vi "save_data.vi"(0 "Experiment Indicator":string, 2 "Date array":string[](array[string]), 3 "Scan direction":i32, 4 "Data Array":dbl[][](array[numeric]), 6 "Username":string, 7 "Stabilisation time (ms)":dbl, 8 "Cell details cluster":T1={"Cell Position"=16, "Cell Label"="", "Pixel to measure"=0, "Area (cm^2)"=0.126, "Variable"="", "Variable value"="", "Scan settings in queue"=0, "Light or dark"="", "Measurement type"=""} {"Pixel to measure" items=["All", "1", "2", "3", "4", "5", "6", "7", "8"]}, 10 "Measurement Delay (ms)":dbl=1.0, 11 "Stabilisation level \n(A or V depending on mode)":dbl=-1.4, 13 "Stabilisation Data":dbl[][](array[numeric])) -> (14 "Master Log":string[][](table), 15 "File path for master log":path, 17 "File path for JV data":path, 18 "File path for JV image":path)   [LabVIEW 2016]
uses:
  <vilib>/Utility/file.llb/Write Delimited Spreadsheet (string).vi
  <vilib>/Utility/file.llb/Read Delimited Spreadsheet (string).vi
  <vilib>/Analysis/NI_AALPro.lvlib
panel:
  out "Vmp":dbl
  out "PCE":dbl
  out "FF":dbl
  out "Voc":dbl
  out "Jsc":dbl
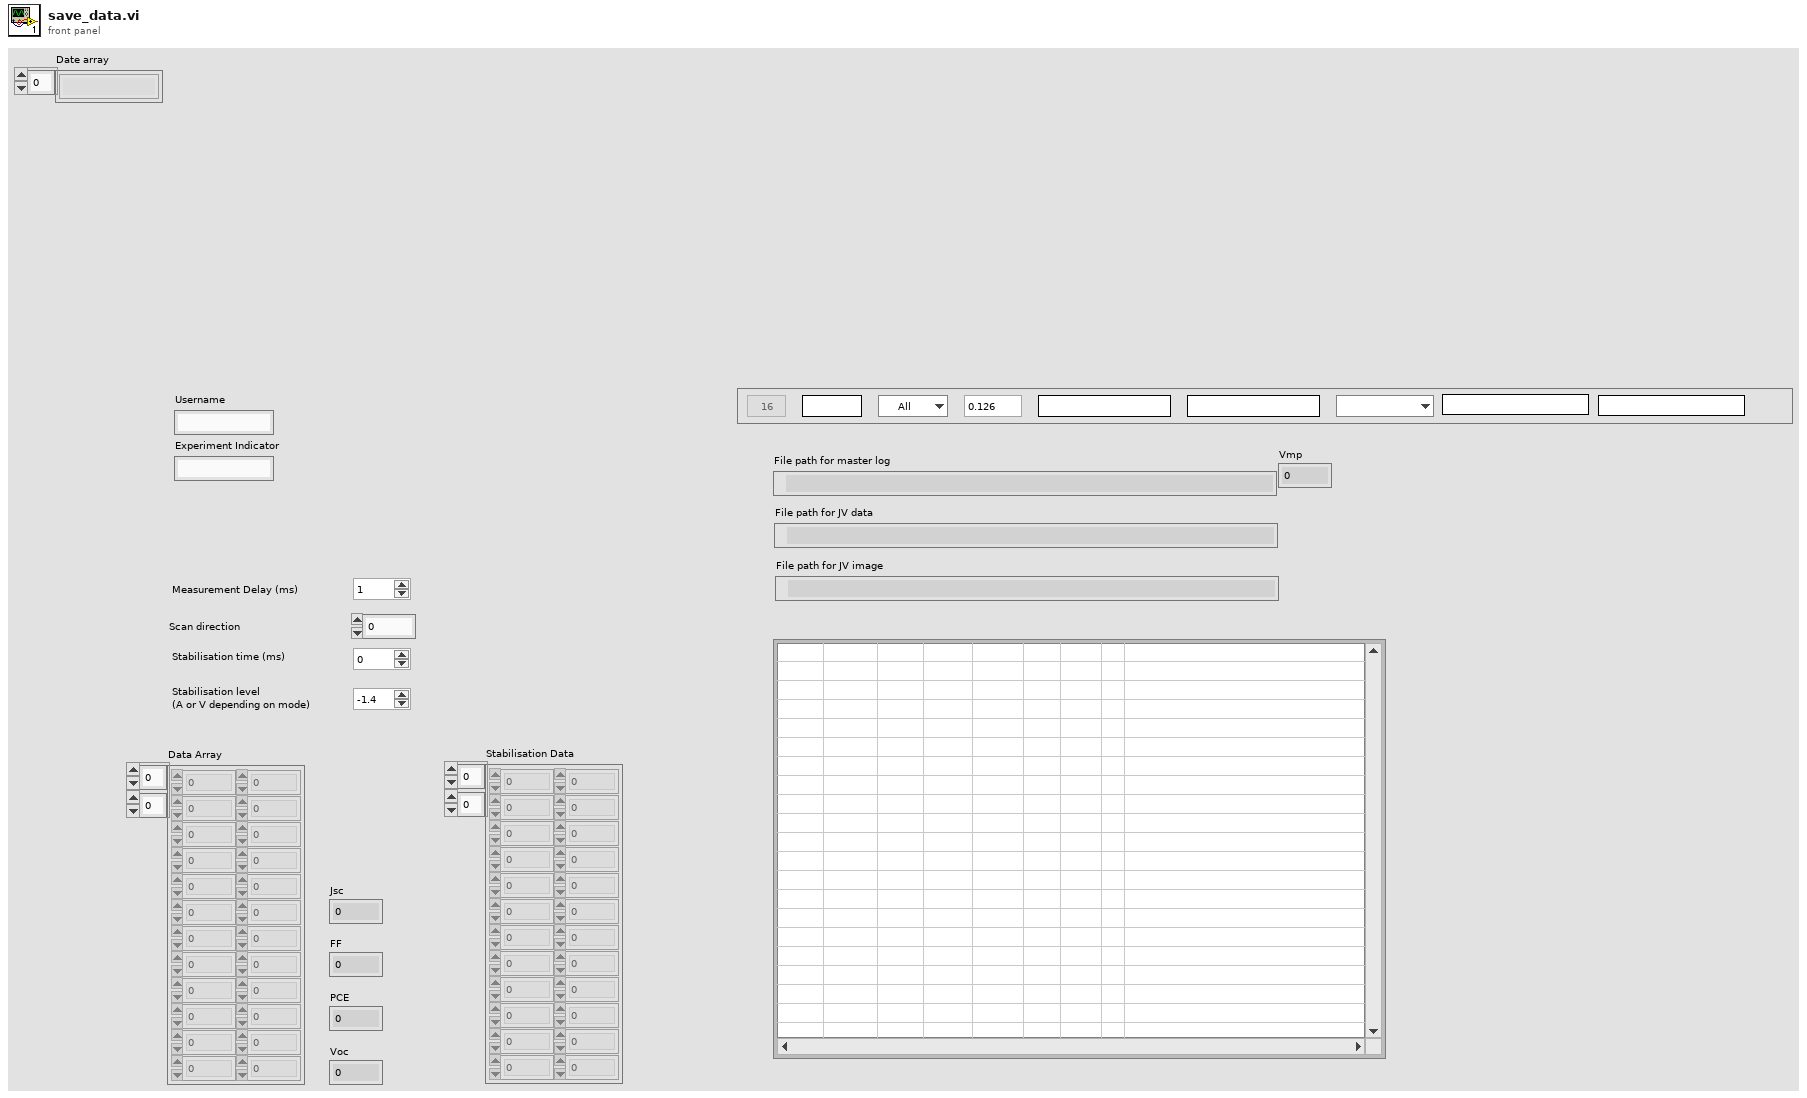
[diagram p1: front panel]
types:
  T1 = cluster{"Cell Position":i32, "Cell Label":string, "Pixel to measure":u16, "Area (cm^2)":dbl, "Variable":string, "Variable value":string, "Scan settings in queue":u16, "Light or dark":string, "Measurement type":string}
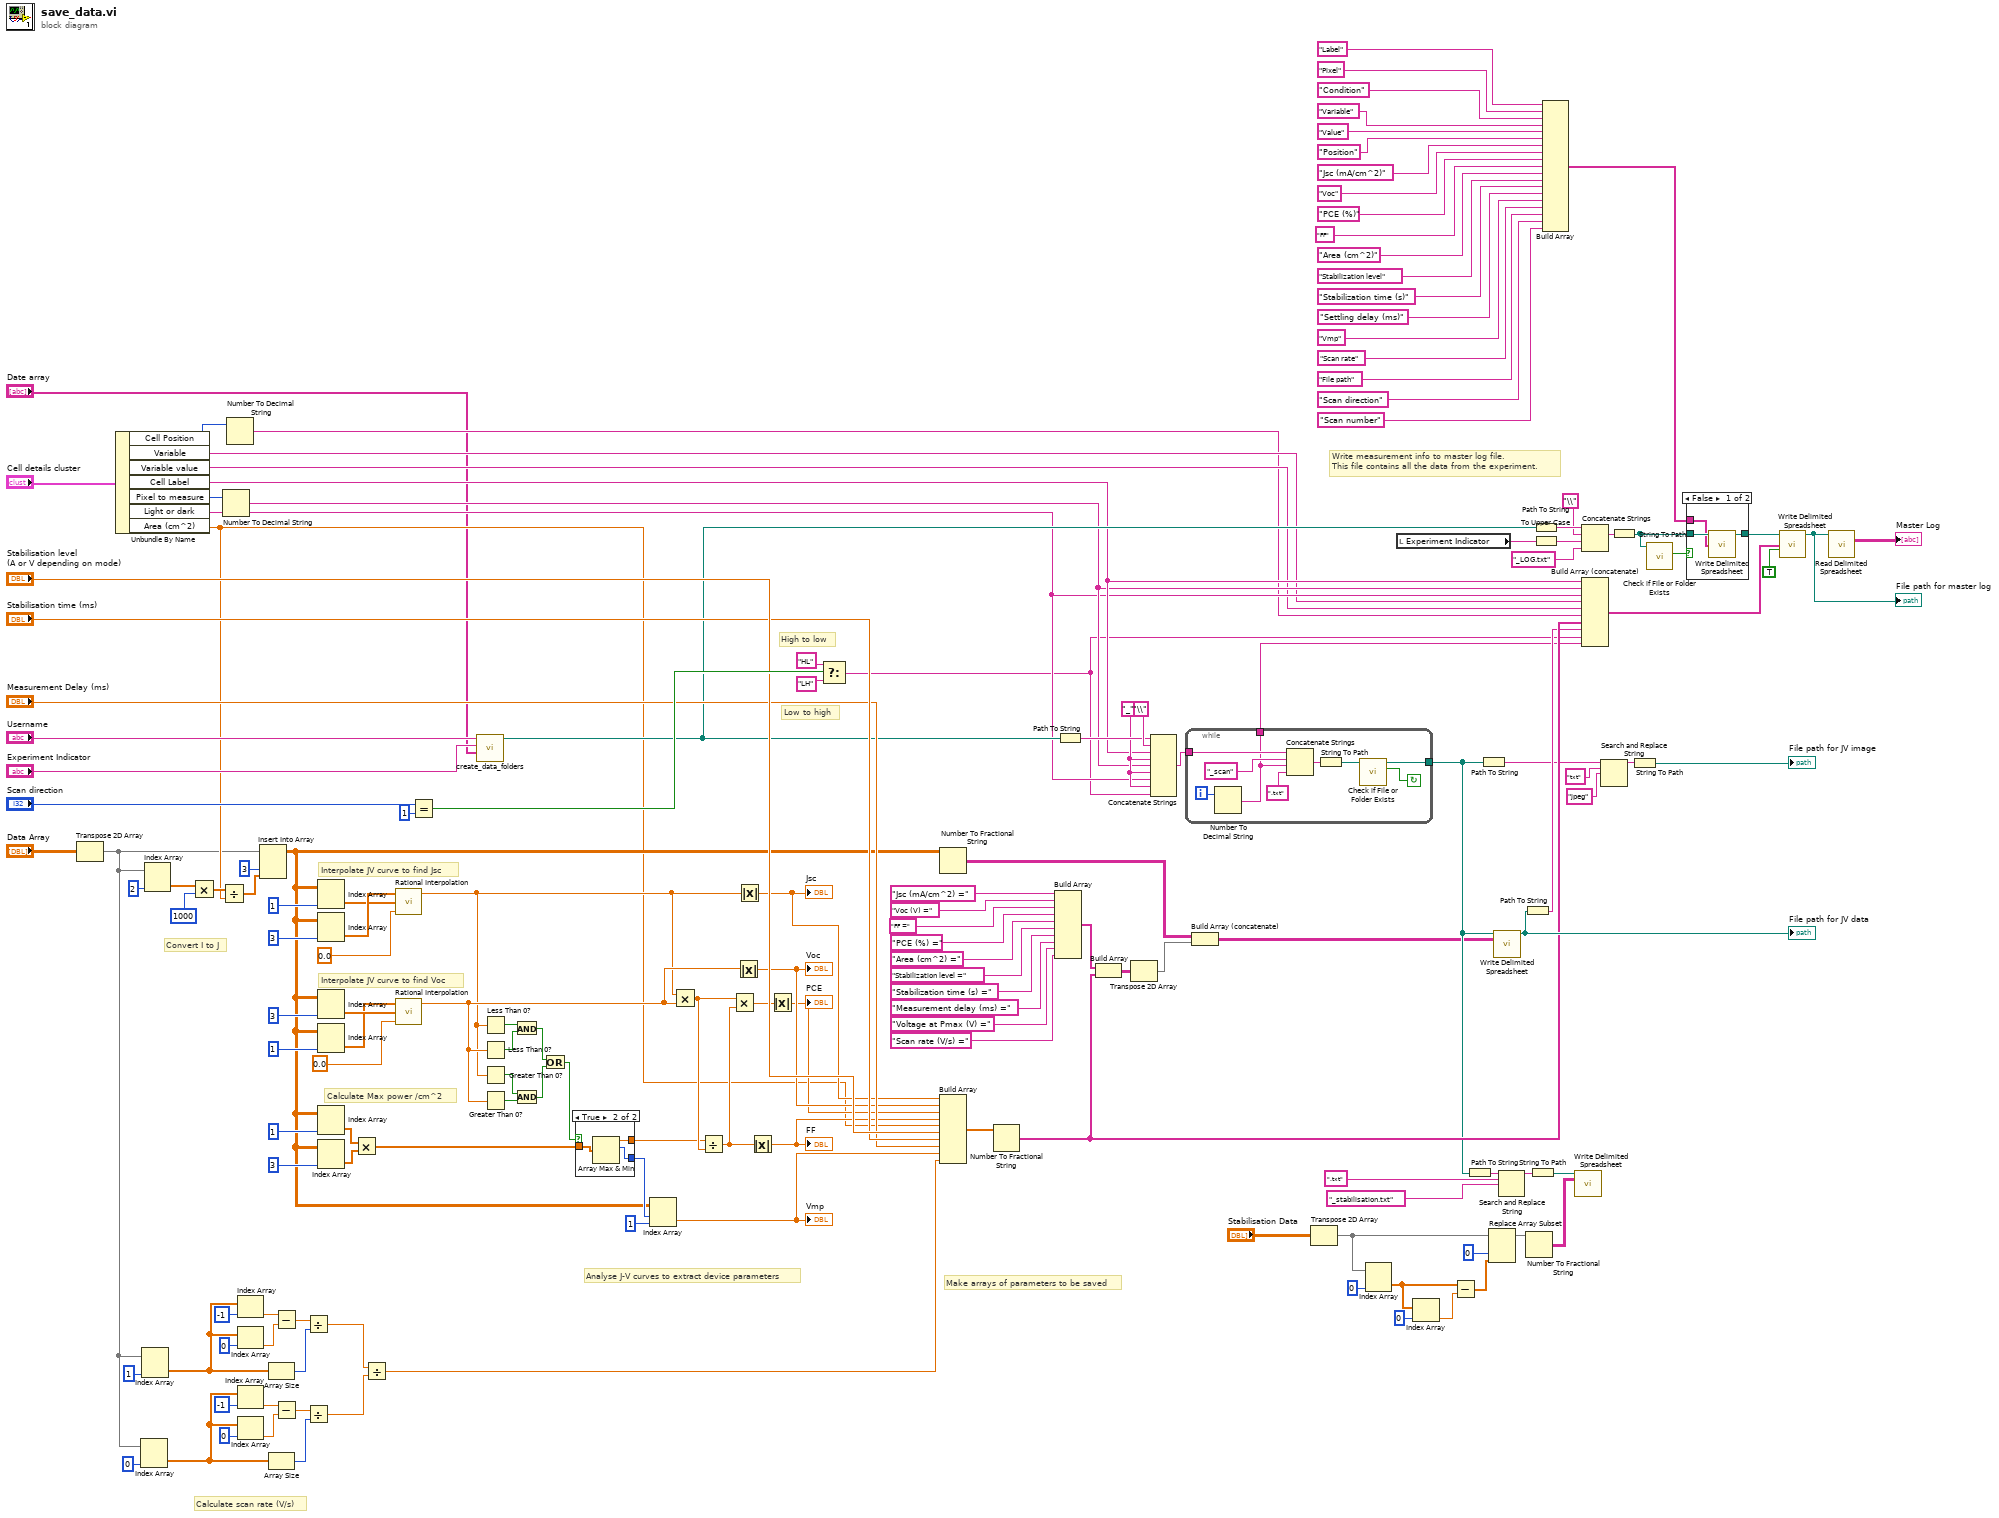
[diagram p0: block diagram]
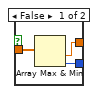
[diagram p3: hidden frame]
diagram:
  w83 = "_"
  # "Calculate scan rate (V/s)"
  # "Convert I to J"
  # "Make arrays of parameters to be saved"
  # "Calculate Max power /cm^2"
  # "Interpolate JV curve to find Voc"
  # "Interpolate JV curve to find Jsc"
  # "Analyse J-V curves to extract device parameters"
  # "Write measurement info to master log file.\nThis file contains all the data from the experiment."
  # "Low to high"
  # "High to low"
  n1 = Transpose 2D Array(2D array="Data Array") -> (transposed array=w27:dbl[][])
  n2 = Unbundle By Name("Cell details cluster") -> ("Cell Position"=w68:i32, "Variable"=w64:string, "Variable value"=w63:string, "Cell Label"=w67:string, "Pixel to measure"=w69:u16, "Light or dark"=w65:string, "Area (cm^2)"=w70:dbl)
  n3 = Index Array(array=w27, index (col)=0 ("disabled index (col)")) -> (element=w20:dbl[])  [unwired: 1 in]
  n4 = Index Array(array=w27, index (col)=1 ("disabled index (col)")) -> (element=w11:dbl[])  [unwired: 1 in]
  n5 = Index Array(array=w27, index (col)=2) -> (element=w88:dbl[])  [unwired: 1 in]
  n6 = Multiply(x=w88, y=1000) -> (x*y=w86:dbl[])
  n7 = Divide(x=w86, y=w70) -> (x/y=w85:dbl[])
  n8 = Number To Decimal String(number=w69) -> (decimal integer string=w66:string)  [unwired: 1 in]
  n9 = Number To Decimal String(number=w68) -> (decimal integer string=w62:string)  [unwired: 1 in]
  n10 = Index Array(array=w11, index=-1) -> (element=w15:dbl)
  n11 = Index Array(array=w11, index=0) -> (element=w14:dbl)
  n12 = Index Array(array=w20, index=-1) -> (element=w22:dbl)
  n13 = Index Array(array=w20, index=0) -> (element=w21:dbl)
  n14 = Insert Into Array(array=w27, index (col)=3, new element=w85) -> (w73:dbl[][])  [unwired: 1 in]
  n15 = Array Size(array=w11) -> (size(s)=w12:i32)
  n16 = Array Size(array=w20) -> (size(s)=w18:i32)
  n17 = Subtract(x=w15, y=w14) -> (x-y=w13:dbl)
  n18 = Subtract(x=w22, y=w21) -> (x-y=w19:dbl)
  n19 = Divide(x=w13, y=w12) -> (x/y=w10:dbl)
  n20 = Divide(x=w19, y=w18) -> (x/y=w9:dbl)
  n21 = Index Array(array=w73, index (col)=1) -> (element=w153:dbl[])  [unwired: 1 in]
  n22 = Index Array(array=w73, index (col)=3) -> (element=w154:dbl[])  [unwired: 1 in]
  n23 = Index Array(array=w73, index (col)=3) -> (element=w152:dbl[])  [unwired: 1 in]
  n24 = Index Array(array=w73, index (col)=1) -> (element=w150:dbl[])  [unwired: 1 in]
  n25 = Index Array(array=w73, index (col)=1) -> (element=w158:dbl[])  [unwired: 1 in]
  n26 = Index Array(array=w73, index (col)=3) -> (element=w157:dbl[])  [unwired: 1 in]
  n27 = Multiply(x=w158, y=w157) -> (x*y=w151:dbl[])
  n28 = Divide(x=w10, y=w9) -> (x/y=w7:dbl)
  n29 = call <vilib>:"Rational Interpolation.vi"("x value"=0.0, "X"=w153, "Y"=w154) -> ("interpolation value"=w87:dbl)  [unwired: 2 out]
  n30 = call <vilib>:"Rational Interpolation.vi"("x value"=0.0, "X"=w152, "Y"=w150) -> ("interpolation value"=w96:dbl)  [unwired: 2 out]
  n31 = Equal?(x="Scan direction", y=1) -> (x = y?=w120:bool)
  n32 = call "create_data_folders.vi"("Date array"="Date array", "Experiment Indicator"="Experiment Indicator", "username"="Username") -> ("Data Output Folder"=w111:path)  [unwired: 8 in]
  n33 = Less Than 0?(x=w87) -> (x < 0?=w102:bool)
  n34 = Less Than 0?(x=w96) -> (x < 0?=w99:bool)
  n35 = Greater Than 0?(x=w87) -> (x > 0?=w100:bool)
  n36 = Greater Than 0?(x=w96) -> (x > 0?=w101:bool)
  n37 = And(x=w102, y=w99) -> (x .and. y?=w104:bool)
  n38 = And(x=w100, y=w101) -> (x .and. y?=w103:bool)
  n39 = Or(x=w104, y=w103) -> (x .or. y?=w98:bool)
  n40 = case shown="True" w98 {
    tunnel: [w166 w170] -> w84
    tunnel: w151 -> [w167 w169]
    tunnel: [w165 w168] -> w74
    frame False {
      n41 = Array Max & Min(array=w167) -> (min value=w166:dbl, min index (indices)=w165:i32)  [unwired: 2 out]
    }
    frame True {
      n42 = Array Max & Min(array=w169) -> (max value=w170:dbl, max index (indices)=w168:i32)  [unwired: 2 out]
    }
  }
  n43 = Index Array(array=w73, index (row)=w74, index (col)=1) -> (element=w71:dbl)
  "Vmp" <- w71
  n44 = Multiply(x=w87, y=w96) -> (x*y=w149:dbl)
  n45 = Divide(x=w84, y=w149) -> (x/y=w92:dbl)
  n46 = Multiply(x=w149, y=w92) -> (x*y=w94:dbl)
  n47 = Absolute Value(x=w96) -> (abs(x)=w95:dbl)
  "Voc" <- w95
  n48 = Absolute Value(x=w87) -> (abs(x)=w97:dbl)
  "Jsc" <- w97
  n49 = Absolute Value(x=w92) -> (abs(x)=w91:dbl)
  "FF" <- w91
  n50 = Absolute Value(x=w94) -> (abs(x)=w93:dbl)
  "PCE" <- w93
  n51 = Select(t="HL", s=w120, f="LH") -> (s? t:f=w2:string)
  n52 = Number To Fractional String(number=w73) -> (F-format string=w122:string[][])  [unwired: 3 in]
  n53 = Build Array(w97, w95, w93, w91, w70, "Stabilisation level \n(A or V depending on mode)", "Stabilisation time (ms)", "Measurement Delay (ms)", w71, w7) -> (w144:dbl[])
  n54 = Number To Fractional String(number=w144) -> (F-format string=w112:string[])  [unwired: 3 in]
  n55 = Build Array("Jsc (mA/cm^2) =", "Voc (V) =", "FF =", "PCE (%) =", "Area (cm^2) =", "Stabilization level =", "Stabilization time (s) =", "Measurement delay (ms) =", "Voltage at Pmax (V) =", "Scan rate (V/s) =") -> (w143:string[])
  n56 = Path To String(path=w111) -> (string=w131:string)
  n57 = Build Array(w143, w112) -> (w140:string[][])
  n58 = Transpose 2D Array(2D array=w140) -> (transposed array=w139:string[][])
  n59 = Concatenate Strings(w131, "\\", w67, w83, w66, w83, w65, w83, w2) -> (w109:string)
  n60 = while {
    tunnel: w109 -> [w179]
    tunnel: [w172] -> w81
    tunnel: [w171] -> w1
    i -> [w177]
    stop <- w173 continue-if-true
    n61 = Number To Decimal String(number=w177) -> (decimal integer string=w171:string)  [unwired: 1 in]
    n62 = Concatenate Strings(w179, "_scan", w171, ".txt") -> (w174:string)
    n63 = String To Path(string=w174) -> (path=w175:path)
    n64 = call <vilib>:"Check if File or Folder Exists.vi"("path"=w175) -> ("file or folder exists?"=w173:bool, "dup path"=w172:path)  [unwired: 8 in, 1 out]
  }
  n65 = Build Array (concatenate)(w122, w139) -> (w41:string[][])
  n66 = Transpose 2D Array(2D array="Stabilisation Data") -> (transposed array=w32:dbl[][])
  n67 = Index Array(array=w32, index (col)=0 ("disabled index (col)")) -> (element=w34:dbl[])  [unwired: 1 in]
  n68 = local read "Experiment Indicator"() -> (w105:string)
  n69 = Index Array(array=w34, index=0) -> (element=w33:dbl)
  n70 = Subtract(x=w34, y=w33) -> (x-y=w30:dbl[])
  n71 = Path To String(path=w81) -> (string=w80:string)
  n72 = Path To String(path=w81) -> (string=w108:string)
  n73 = Replace Array Subset(array=w32, new element=w30, index (col)=0 ("disabled index (col)")) -> (w29:dbl[][])  [unwired: 1 in]
  n74 = call-poly <vilib>:"Write Delimited Spreadsheet.vi"("file path (dialog if empty)"=w81, "2D data"=w41) -> ("new file path (Not A Path if cancelled)"=w118:path)  [unwired: 12 in, 1 out]
  "File path for JV data" <- w118
  n75 = Search and Replace String(input string=w80, search string=".txt", replace string="_stabilisation.txt") -> (result string=w77:string)  [unwired: 5 in, 3 out]
  n76 = Path To String(path=w118) -> (string=w110:string)
  n77 = Number To Fractional String(number=w29) -> (F-format string=w42:string[][])  [unwired: 3 in]
  n78 = String To Path(string=w77) -> (path=w76:path)
  n79 = Path To String(path=w111) -> (string=w135:string)
  n80 = To Upper Case(1:w105) -> (0:w106:string)
  n81 = Build Array("Label", "Pixel", "Condition", "Variable", "Value", "Position", "Jsc (mA/cm^2)", "Voc", "PCE (%)", "FF", "Area (cm^2)", "Stabilization level", "Stabilization time (s)", "Settling delay (ms)", "Vmp", "Scan rate", "File path", "Scan direction", "Scan number") -> (w43:string[])
  n82 = call-poly <vilib>:"Write Delimited Spreadsheet.vi"("file path (dialog if empty)"=w76, "2D data"=w42) -> ()  [unwired: 12 in, 2 out]
  n83 = Concatenate Strings(w135, "\\", w106, "_LOG.txt") -> (w133:string)
  n84 = Build Array (concatenate)(w67, w66, w65, w64, w63, w62, w112, w110, w2, w1) -> (w40:string[])
  n85 = Search and Replace String(input string=w108, search string="txt", replace string="jpeg") -> (result string=w130:string)  [unwired: 5 in, 3 out]
  n86 = String To Path(string=w133) -> (path=w45:path)
  n87 = String To Path(string=w130) -> (path=→"File path for JV image":path)
  n88 = call <vilib>:"Check if File or Folder Exists.vi"("path"=w45) -> ("file or folder exists?"=w46:bool)  [unwired: 8 in, 2 out]
  n89 = case shown="False" w46 {
    tunnel: w45 -> [w182 w183]
    tunnel: [w181 w183] -> w44
    tunnel: w43 -> [w180 _]
    frame False {
      n90 = call-poly <vilib>:"Write Delimited Spreadsheet.vi"("file path (dialog if empty)"=w182, "1D data"=w180) -> ("new file path (Not A Path if cancelled)"=w181:path)  [unwired: 12 in, 1 out]
    }
    frame True {
    }
  }
  n91 = call-poly <vilib>:"Write Delimited Spreadsheet.vi"("file path (dialog if empty)"=w44, "1D data"=w40, "append to file? (new file:F)"=TRUE) -> ("new file path (Not A Path if cancelled)"=w125:path)  [unwired: 11 in, 1 out]
  "File path for master log" <- w125
  n92 = call-poly <vilib>:"Read Delimited Spreadsheet.vi"("file path (dialog if empty)"=w125) -> ("all rows"=→"Master Log":string[][])  [unwired: 9 in, 5 out]
